vi "osa_get sensor toggle command string.vi"(11 "OSB status/control":refnum<vi>) -> (0 "status string":string, 2 "command string 2":string[](array[string]), 3 "command string 1":string[](array[string]))   [LabVIEW 2021]
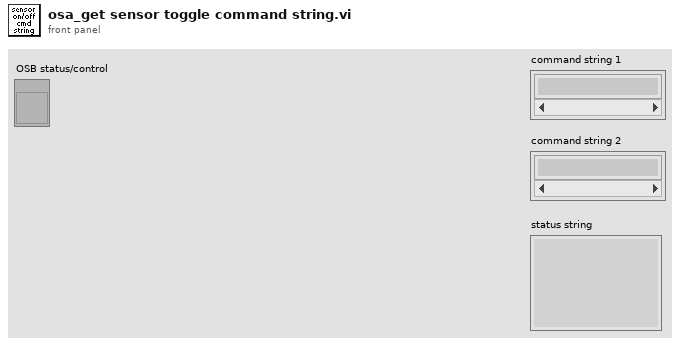
[diagram p1: front panel]
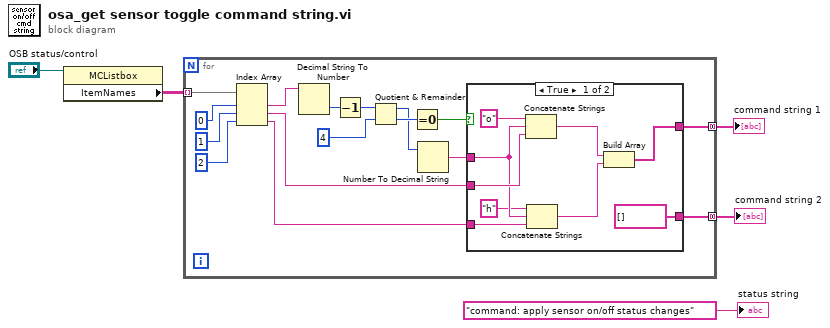
[diagram p0: block diagram]
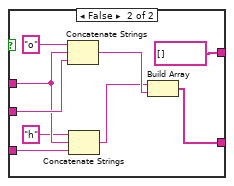
[diagram p2: hidden frame]
diagram:
  n1 = property class="MCListbox"(reference="OSB status/control") -> ("ItemNames"=w4:string[][])  [unwired: 1 in, 2 out]
  n2 = for {
    tunnel: w4 -> [w21] mode=indexing
    tunnel: [w10] -> w3 mode=concatenating
    tunnel: [w9] -> w2 mode=concatenating
    n3 = Index Array(array=w21, index #1=0 ("index"), index #2=1 ("index"), index #3=2 ("index")) -> (element #1=w17:string, element #2=w12:string, element #3=w11:string)
    n4 = Decimal String To Number(string=w17) -> (number=w7:i32)  [unwired: 2 in, 1 out]
    n5 = Decrement(x=w7) -> (x-1=w6:i32)
    n6 = Quotient & Remainder(x=w6, y=4) -> (x-y*floor(x/y)=w8:i32, floor(x/y)=w15:i32)
    n7 = Equal To 0?(x=w15) -> (x = 0?=w14:bool)
    n8 = Number To Decimal String(number=w8) -> (decimal integer string=w13:string)  [unwired: 1 in]
    n9 = case shown="True" w14 {
      tunnel: w13 -> [w27 w36]
      tunnel: w12 -> [w29 w38]
      tunnel: w11 -> [w28 w37]
      tunnel: [w24 string[] []] -> w10
      tunnel: [string[] [] w33] -> w9
      frame True {
        n10 = Concatenate Strings("o", w27, w29) -> (w23:string)
        n11 = Concatenate Strings("h" ("string"), w27, w28) -> (w22:string)
        n12 = Build Array(w23, w22) -> (w24:string[])
      }
      frame False {
        n13 = Concatenate Strings("o", w36, w38) -> (w34:string)
        n14 = Concatenate Strings("h" ("string"), w36, w37) -> (w31:string)
        n15 = Build Array(w31, w34) -> (w33:string[])
      }
    }
  }
  "command string 1" <- w3
  "command string 2" <- w2
  "status string" <- "command: apply sensor on/off status changes" ("status string")
